vi "CRYISO Freq.vi"(3 "Lower Freq":dbl=100.0 format="%.2f", 4 "ISO series":u16(ring) items=["R10 (1/3 Oct.)", "R20 (1/6 Oct.)", "R40 (1/12 Oct.)", "R80 (1/24 Oct.)", "1/1 Octave"], 5 "Higher Freq":dbl=6310.0 format="%.2f") -> (0 "Lower ISO Freq":dbl=100.0 format="%.2f", 1 "No. Steps":i32=20, 2 "Higher ISO Freq":dbl=8000.0 format="%.2f")   [LabVIEW 2013]
uses:
  CRYStimulus Global.vi
panel:
  # "This VI finds the nearest ISO frequency\nto the input frequency in the chosen series."
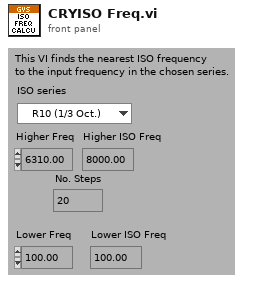
[diagram p1: front panel]
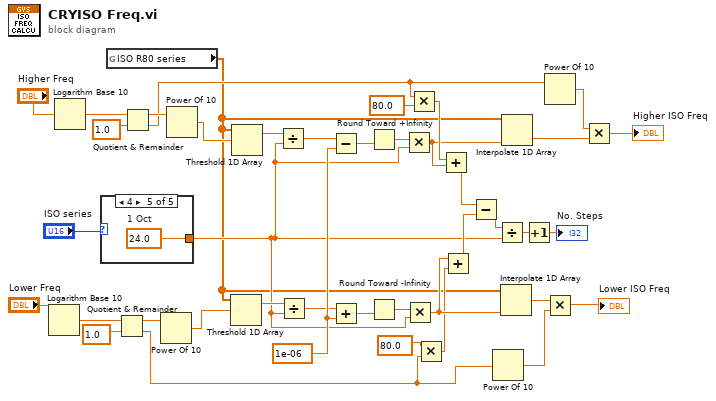
[diagram p0: block diagram]
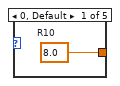
[diagram p2: hidden frame]
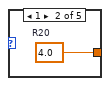
[diagram p3: hidden frame]
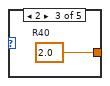
[diagram p4: hidden frame]
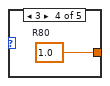
[diagram p5: hidden frame]
diagram:
  w7 = 1e-06
  n1 = Logarithm Base 10(1:"Lower Freq") -> (0:w30:dbl)
  n2 = Logarithm Base 10(1:"Higher Freq") -> (0:w20:dbl)
  n3 = case shown="4" "ISO series" {
    tunnel: [w42 w43 w44 w45 w46] -> w2
    frame 0, Default {
      w42 = 8.0  # R10
    }
    frame 1 {
      w43 = 4.0  # R20
    }
    frame 2 {
      w44 = 2.0  # R40
    }
    frame 3 {
      w45 = 1.0  # R80
    }
    frame 4 {
      w46 = 24.0  # 1 Oct
    }
  }
  n4 = global read "CRYStimulus Global.vi" "ISO R80 series"() -> (w1:dbl[])
  n5 = Quotient & Remainder(x=w30, y=1.0) -> (x-y*floor(x/y)=w23:dbl, floor(x/y)=w24:dbl)
  n6 = Quotient & Remainder(x=w20, y=1.0) -> (x-y*floor(x/y)=w19:dbl, floor(x/y)=w13:dbl)
  n7 = Power Of 10(x=w23) -> (10^x=w29:dbl)
  n8 = Power Of 10(x=w19) -> (10^x=w17:dbl)
  n9 = Threshold 1D Array(2:w29, 3:w1) -> (0:w37:dbl)  [unwired: 1 out]
  n10 = Threshold 1D Array(2:w17, 3:w1) -> (0:w40:dbl)  [unwired: 1 out]
  n11 = Divide(x=w40, y=w2) -> (x/y=w5:dbl)
  n12 = Divide(x=w37, y=w2) -> (x/y=w6:dbl)
  n13 = Subtract(x=w5, y=w7) -> (x-y=w4:dbl)
  n14 = Add(x=w6, y=w7) -> (x+y=w3:dbl)
  n15 = Round Toward +Infinity(x=w4) -> (ceil(x): smallest int >= x=w39:dbl)
  n16 = Round Toward -Infinity(1:w3) -> (0:w38:dbl)
  n17 = Multiply(x=w39, y=w2) -> (x*y=w11:dbl)
  n18 = Multiply(x=w38, y=w2) -> (x*y=w33:dbl)
  n19 = Multiply(x=w13, y=80.0) -> (x*y=w12:dbl)
  n20 = Multiply(x=80.0, y=w24) -> (x*y=w25:dbl)
  n21 = Add(x=w12, y=w11) -> (x+y=w10:dbl)
  n22 = Add(x=w33, y=w25) -> (x+y=w22:dbl)
  n23 = Subtract(x=w10, y=w22) -> (x-y=w27:dbl)
  n24 = Power Of 10(x=w24) -> (10^x=w28:dbl)
  n25 = Divide(x=w27, y=w2) -> (x/y=w35:dbl)
  n26 = Interpolate 1D Array(1:w33, 2:w1) -> (0:w36:dbl)
  n27 = Interpolate 1D Array(1:w11, 2:w1) -> (0:w15:dbl)
  n28 = Increment(x=w35) -> (x+1=→"No. Steps":dbl)
  n29 = Power Of 10(x=w13) -> (10^x=w16:dbl)
  n30 = Multiply(x=w36, y=w28) -> (x*y=→"Lower ISO Freq":dbl)
  n31 = Multiply(x=w16, y=w15) -> (x*y=→"Higher ISO Freq":dbl)
